vi "GetCallerVIName.vi"() -> (3 "VI name":string)   [LabVIEW 2017, in "Communication.lvlib"]
uses:
  Communication.lvlib
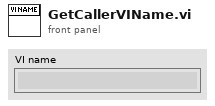
[diagram p1: front panel]
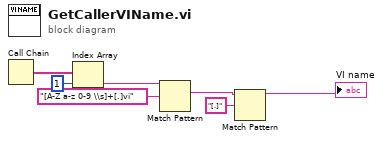
[diagram p0: block diagram]
diagram:
  n1 = Call Chain() -> (call chain=w7:string[])
  n2 = Index Array(array=w7, index=1) -> (element=w6:string)
  n3 = Match Pattern(string=w6, regular expression="[A-Z a-z 0-9 \\s]+[.]vi") -> (match substring=w3:string)  [unwired: 1 in, 3 out]
  n4 = Match Pattern(string=w3, regular expression="[.]") -> (before substring=→"VI name":string)  [unwired: 1 in, 3 out]
